vi "Generate File Name.vi"(5 "slice":i32, 7 "tile":i32) -> (4 "appended path":path)   [LabVIEW 2018]
uses:
  General/Controls/FGV Actions.ctl
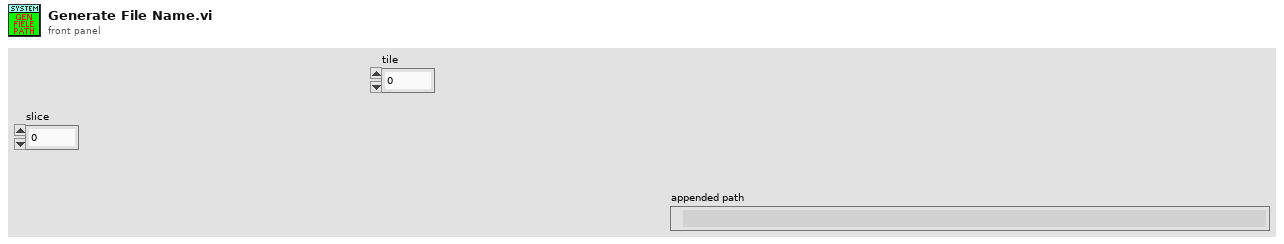
[diagram p1: front panel]
types:
  T1 = enum16{"File name", "X stage", "Y stage", "Slice plane", "Image plane", "time", "output"}
  T2 = typedef "FGV Actions.ctl" = enum16{"Init", "Set", "Get", "Clear"}
  T3 = typedef "System Parameters.ctl" = cluster{"Optical Parameters":T4, "Vibratome":T5, "Table Stages":T6, "Imaging Parameter":T9, "Galvo HW Parameters":cluster{"Analog Out Channel":tag, "Min Voltage":dbl, "Max Voltage":dbl, "Pixel Clock Source":tag, "Sample Rate":dbl, "Line Clock Out Ch":tag, "2P ready check":tag}, "Alazar parameters":T11, "Mosaic Paramter":T18, "Manual Controls":T19, "Z stage setting":T23, "Attenuator":T24, "Pause?":bool}
  T4 = typedef "Optical Parameters.ctl" = cluster{"Obj. Focal Length [mm]":dbl, "Scan Lens EFL[mm]":dbl, "Tube Lens EFL[mm]":dbl, "Galvo V Range (+/-)":dbl, "Galvo Max Half Angle [Deg]":dbl, "Max Galvo Range[%]":dbl}
  T5 = typedef "Vibratome Parameters.ctl" = cluster{"Pre Cut Dwell [s]":dbl, "Blade Frequency [RPM]":u16, "Slice Speed [mm/s]":dbl, "Post Cut Dwell [s]":dbl, "Ramp Time [s]":dbl, "Start X [mm]":dbl, "Start Y [mm]":dbl, "Slice Length [mm]":dbl, "Slice Axis":enum16{"X Axis", "Y Axis", "Z Axis"}, "Controller VISA Ref":refnum<visa-resource-name>}
  T6 = typedef "Translation Stage Parameters.ctl" = cluster{"X Stage":T7, "Y Stage":T7, "Z Stage":T7, "Attenuator":T7}
  T7 = typedef "Translation Stage Cluster.ctl" = cluster{"Position":dbl, "Is.Enabled?":bool, "Is.Connected?":bool, "Device SN":string, "AccelerationMaximum":dbl, "VelocityMaximum":dbl, "Acceleration":dbl, "Velocity":dbl, "waitTimeout (ms)":i32, "Model":T8, "Is.Homed?":bool, "MOVE":bool}
  T8 = typedef "Translation Stage Types.ctl" = enum16{"None", "Thorlabs LTS", "Thorlabs MLJ"}
  T9 = typedef "Imaging Parameters.ctl" = cluster{"Raster Scan Direction":T10, "Pixel Dwell Time [Clock Cycles]":u16, "Flyback Time [Clock Cycles]":u16, "XY Center [um]":cluster{"X":dbl, "Y":dbl}, "Pixel Step Size [um] X":dbl, "XY Image Size":enum16{"32 x 32", "64 x 64", "128 x 128", "256 x 256", "512 x 512", "1024 x 1024", "2048 x 2048"}, "Custom":bool, "Custom Size":cluster{"X":u16, "Y":u16}, "Line Averages":u16, "Pixel Step Size [um] Y":dbl}
  T10 = typedef "Scan Direction.ctl" = enum16{"Uni Directional", "Bi Directional", "None"}
  T11 = typedef "Alazar parameters.ctl" = cluster{"Trigger Settings":cluster{"General Trigger Settings":T12, "Trigger Engine 1":T13, "Trigger Engine 2":T13}, "Device ID":T14, "Ch A Input Control":T15, "Ch B Input Control":T15, "Acq Settings":T16, "Capture Clock":T17}
  T12 = typedef "General Trigger Settings.ctl" = cluster{"Trigger Operation":u32, "Coupling ID":u32, "Range ID":u32, "Delay":u32, "Timeout Ticks":u32, "Mode":u32, "Parameter":u32}
  T13 = typedef "Trigger Engine Controls.ctl" = cluster{"Trigger Engine":u32, "Source":u32, "Slope":u32, "Level":u32}
  T14 = typedef "Alazar Device ID.ctl" = cluster{"System ID":u32, "Board ID":u32}
  T15 = typedef "Channel Input Controls.ctl" = cluster{"Channel":u8, "Coupling":u32, "Range":u32, "Impedance":u32}
  T16 = typedef "Alazar Acquisition Settings.ctl" = cluster{"Record Length":u32, "Offset":u32, "Records Per Buffer":u32, "Records Count (Records/Acq)":u32, "Window Type":u32, "Footer":u32, "Samples per record":u32, "Output Format":u32}
  T17 = typedef "Clock Controls.ctl" = cluster{"Sample Rate":u32, "Decimation":u32, "Source":u32, "Edge":u32}
  T18 = typedef "Mosaic Parameter.ctl" = cluster{"X Axis":cluster{"Start [mm]":dbl, "Steps [pts]":dbl, "End [mm]":dbl}, "Y Axis":cluster{"Start [mm]":dbl, "Steps [pts]":dbl, "End [mm]":dbl}, "Scan Pattern":enum16{"Uni-directional", "Bi-Directional", "Spiral Out", "Spiral In"}, "Overlap Options":cluster{"Overlap Type":enum16{"No Overlap", "X Only", "Y Only", "X and Y"}, "Percent Overlap":u8, "Justify":enum16{"Start", "Center", "End"}}}
  T19 = typedef "Manual Controls.ctl" = cluster{"Data Path":path, "Save parameters":T20, "Acquisition mode":T21, "PSOCT Channel":u32, "Save data?":bool, "AIP rotation angle":dbl, "Outgoing Mail Server (SMTP)":string, "Email":string, "Password":string, "Carrier 1":enum16{"T-Mobile", "AT&T", "Verizon", "Sprint"}, "phone number 1":string, "Subject":string, "Message":string, "Carrier 2":enum16{"T-Mobile", "AT&T", "Verizon", "Sprint"}, "phone number 2":string, "Outputs for GPU FFT":T22, "First Slice #":i32}
  T20 = typedef "FFT parameters.ctl" = cluster{"start pixel":i32, "#pixels to save":i32}
  T21 = typedef "FFT mode.ctl" = enum16{"ThorOCT B line", "ThorOCT Spectral", "ThorOCT FFT", "Alazar B line", "Alazar FFT", "GPU FFT", "Alazar Spectral", "Simulation", "auto adjust focus", "Save all"}
  T22 = typedef "GPU FFT outputs.ctl" = enum16{"Amp + Phase diff", "Amp + Phase", "Amp only"}
  T23 = typedef "Vibratome Param.ctl" = cluster{"first cut height(mm)":dbl, "cut thickness[um]":u32[], "#cycles":u16, "PSOCT thickness(um)":u32[], "First image height(mm)":dbl, "Pause?":bool[], "Z0":dbl, "fixed Z0?":bool, "Cut_aft_2P?(leave empty if no 2P)":bool[], "2P thickness(um) (leave empty if not used)":u32[], "2P_cover_all_depth? (leave empty if no 2P)":bool[]}
  T24 = typedef "attenuator.ctl" = cluster{"Power after Objective (recalibrate every 6 month)":dbl[]}
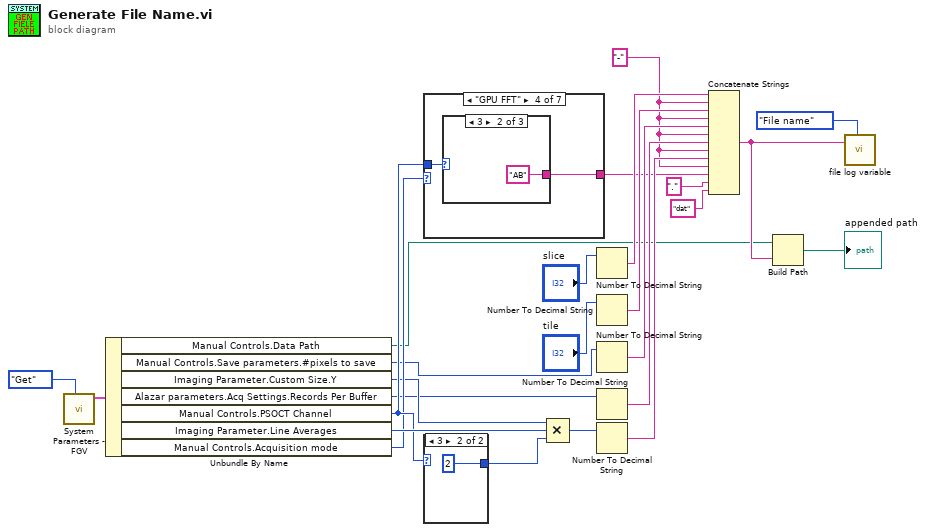
[diagram p0: block diagram]
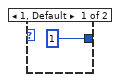
[diagram p2: hidden frame]
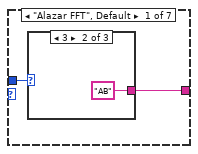
[diagram p3: hidden frame]
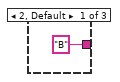
[diagram p4: hidden frame]
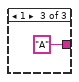
[diagram p5: hidden frame]
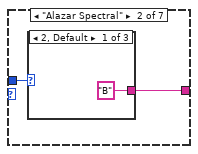
[diagram p6: hidden frame]
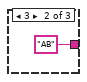
[diagram p7: hidden frame]
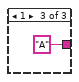
[diagram p8: hidden frame]
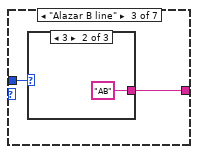
[diagram p9: hidden frame]
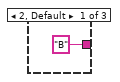
[diagram p10: hidden frame]
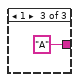
[diagram p11: hidden frame]
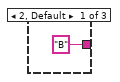
[diagram p12: hidden frame]
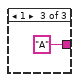
[diagram p13: hidden frame]
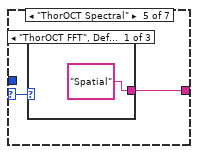
[diagram p14: hidden frame]
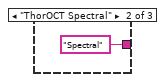
[diagram p15: hidden frame]
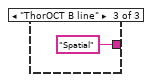
[diagram p16: hidden frame]
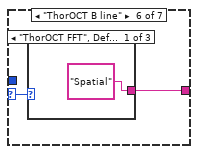
[diagram p17: hidden frame]
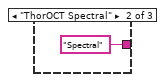
[diagram p18: hidden frame]
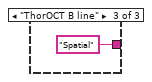
[diagram p19: hidden frame]
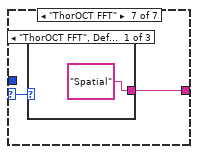
[diagram p20: hidden frame]
diagram:
  w3 = "-" ("string")
  n1 = call "System Parameters - FGV.vi"("Actions"=FGV_Actions."Get") -> ("System Parameters [Out]"=w17:T3)  [unwired: 9 in, 1 out]
  n2 = Unbundle By Name(w17) -> ("Manual Controls.Data Path"=w1:path, "Manual Controls.Save parameters.#pixels to save"=w13:i32, "Imaging Parameter.Custom Size.Y"=w14:u16, "Alazar parameters.Acq Settings.Records Per Buffer"=w12:u32, "Manual Controls.PSOCT Channel"=w16:u32, "Imaging Parameter.Line Averages"=w20:u16, "Manual Controls.Acquisition mode"=w15:T21)
  n3 = case shown="\"GPU FFT\"" w15 {
    selector: w15 -> [_ _ _ _ w46 w51 w56]
    tunnel: [w27 w32 w37 w42 w47 w52 w57] -> w2
    tunnel: w16 -> [w26 w31 w36 w41 _ _ _]
    frame "Alazar FFT", Default {
      n4 = case shown="3" w26 {
        tunnel: ["B" "AB" "A"] -> w27
        frame 2, Default {
        }
        frame 3 {
        }
        frame 1 {
        }
      }
    }
    frame "Alazar Spectral" {
      n5 = case shown="2, Default" w31 {
        tunnel: ["B" "AB" "A"] -> w32
        frame 2, Default {
        }
        frame 3 {
        }
        frame 1 {
        }
      }
    }
    frame "Alazar B line" {
      n6 = case shown="3" w36 {
        tunnel: ["B" "AB" "A"] -> w37
        frame 2, Default {
        }
        frame 3 {
        }
        frame 1 {
        }
      }
    }
    frame "GPU FFT" {
      n7 = case shown="3" w41 {
        tunnel: ["B" "AB" "A"] -> w42
        frame 2, Default {
        }
        frame 3 {
        }
        frame 1 {
        }
      }
    }
    frame "ThorOCT Spectral" {
      n8 = case shown="\"ThorOCT FFT\", Default" w46 {
        tunnel: ["Spatial" "Spectral" "Spatial"] -> w47
        frame "ThorOCT FFT", Default {
        }
        frame "ThorOCT Spectral" {
        }
        frame "ThorOCT B line" {
        }
      }
    }
    frame "ThorOCT B line" {
      n9 = case shown="\"ThorOCT FFT\", Default" w51 {
        tunnel: ["Spatial" "Spectral" "Spatial"] -> w52
        frame "ThorOCT FFT", Default {
        }
        frame "ThorOCT Spectral" {
        }
        frame "ThorOCT B line" {
        }
      }
    }
    frame "ThorOCT FFT" {
      n10 = case shown="\"ThorOCT FFT\", Default" w56 {
        tunnel: ["Spatial" "Spectral" "Spatial"] -> w57
        frame "ThorOCT FFT", Default {
        }
        frame "ThorOCT Spectral" {
        }
        frame "ThorOCT B line" {
        }
      }
    }
  }
  n11 = case shown="3" w16 {
    tunnel: [1 2] -> w19
    frame 1, Default {
    }
    frame 3 {
    }
  }
  n12 = Compound Arithmetic op=MULTIPLY(w14, w20, w19) -> (w11:i32)
  n13 = Number To Decimal String(number="slice") -> (decimal integer string=w8:string)  [unwired: 1 in]
  n14 = Number To Decimal String(number="tile") -> (decimal integer string=w7:string)  [unwired: 1 in]
  n15 = Number To Decimal String(number=w13) -> (decimal integer string=w6:string)  [unwired: 1 in]
  n16 = Number To Decimal String(number=w12) -> (decimal integer string=w5:string)  [unwired: 1 in]
  n17 = Number To Decimal String(number=w11) -> (decimal integer string=w4:string)  [unwired: 1 in]
  n18 = Concatenate Strings(w8, w3, w7, w3, w6, w3, w5, w3, w4, w3, w2, "." ("string"), "dat" ("string")) -> (w9:string)
  n19 = Build Path(base path=w1, name or relative path=w9) -> (appended path=→"appended path":path)
  n20 = call "file log variable.vi"("file name"=w9, "Item"=T1."File name") -> ()  [unwired: 16 in, 2 out]
